vi "Configure Library Classes in Memory for Build.vi"(5 "custom class options":T1[](array[typedef]), 7 "target name (My Computer)":string="My Computer", 9 "enable debug? (F)":bool, 10 "save VIs? (T)":bool=TRUE, 11 "library name":string="DSF Core.lvlib") -> (0 "error out":errorcluster)   [LabVIEW 2017, in "Build Automation.lvlib"]
uses:
  Build Automation.lvlib
  Class VI Options.ctl
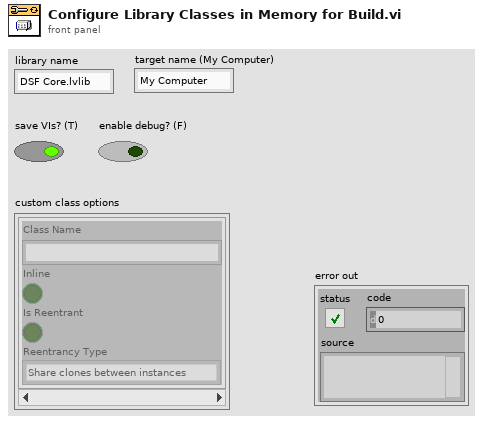
[diagram p1: front panel]
types:
  T1 = typedef "Build Automation.lvlib/Class VI Options.ctl" = cluster{"Class Name":string, "Inline":bool, "Is Reentrant":bool, "Reentrancy Type":enum16{"Share clones between instances", "Preallocate clone for each instance"}}
  T2 = cluster{"Status Message":refnum<data-value>, "Progress":refnum<data-value>, "Stop":refnum<data-value>}
  T3 = enum16{"Share clones between instances", "Preallocate clone for each instance"}
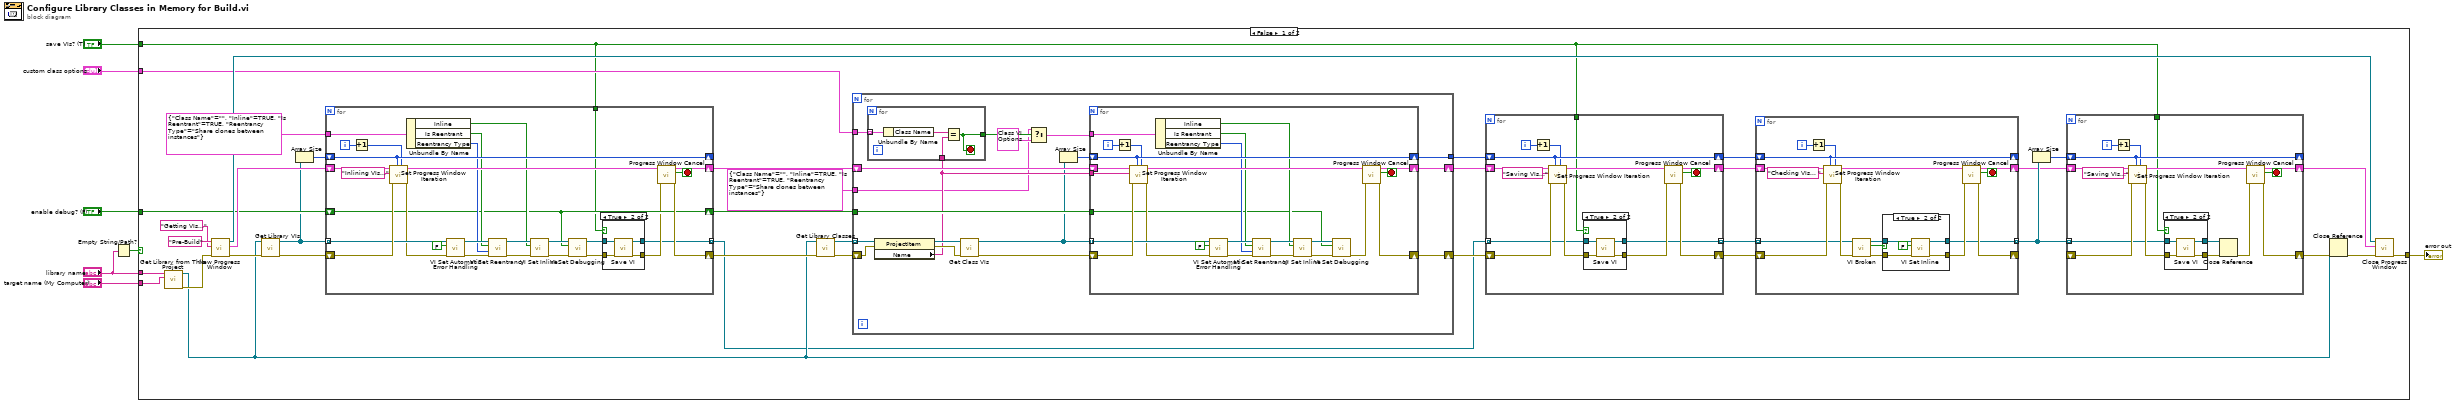
[diagram p0: block diagram]
diagram:
  n1 = Empty String/Path?(string/path="library name") -> (empty?=w6:bool)
  n2 = case shown="False" w6 {
    tunnel: [w43 _] -> w4
    tunnel: "enable debug? (F)" -> [w25 _]
    tunnel: "library name" -> [w38 _]
    tunnel: "save VIs? (T)" -> [w8 _]
    tunnel: "target name (My Computer)" -> [w36 _]
    tunnel: "custom class options" -> [w23 _]
    frame False {
      n3 = call "Get Library from This Project.vi"("Target Name (My Computer)"=w36, "Library Name"=w38) -> ("error out"=w37:errorcluster, "Library Refnum"=w27:refnum<vi>)  [unwired: 8 in]
      n4 = call "New Progress Window.vi"("error in (no error)"=w37, "Initial Message"="Getting VIs...", "Window Title"="Pre-Build" ("WindowTitle")) -> ("error out"=w28:errorcluster, "DVRs"=w29:T2, "VI refnum"=w44:refnum<vi>)  [unwired: 6 in]
      n5 = call "Get Library VIs.vi"("error in (no error)"=w28, "library ref"=w27) -> ("error out"=w26:errorcluster, "vi refs"=w21:refnum<vi>[])  [unwired: 8 in]
      n6 = Array Size(array=w21) -> (size(s)=w22:i32)
      n7 = for {
        tunnel: w21 -> [w64] mode=indexing
        shift-right: [w71] -> w31
        shift-left: w29 -> [w68]
        shift-right: [w65] -> w30
        shift-left: w26 -> [w66]
        tunnel: [w45] -> w11 mode=indexing
        shift-right: [w63] -> _
        shift-left: w22 -> [w63]
        tunnel: T1 {"Class Name"="", "Inline"=TRUE, "Is Reentrant"=TRUE, "Reentrancy Type"=enum."Share clones between instances"} ("f") -> [w56]
        shift-right: [w51] -> w24
        shift-left: w25 -> [w51]
        tunnel: w8 -> [w46]
        i -> [w73]
        stop <- w72 stop-if-true
        n8 = Increment(x=w73) -> (x+1=w62:i32)
        n9 = call "Set Progress Window Iteration.vi"("current iteration"=w62, "total iterations"=w63, "error in (no error)"=w66, "Status Message"="Inlining VIs...", "DVRs in"=w68) -> ("error out"=w53:errorcluster, "DVRs out"=w67:T2)  [unwired: 5 in]
        n10 = Unbundle By Name(w56) -> ("Inline"=w55:bool, "Is Reentrant"=w54:bool, "Reentrancy Type"=w52:T3)
        n11 = call "VI Set Automatic Error Handling.vi"("error in (no error)"=w53, "Automatic Error Handling"=FALSE, "vi ref in"=w64) -> ("error out"=w57:errorcluster, "vi ref out"=w69:refnum<vi>)  [unwired: 7 in]
        n12 = call "VI Set Reentrancy.vi"("error in (no error)"=w57, "Reentrancy Type (shared clone)"=w52, "Is Reentrant"=w54, "vi ref in"=w69) -> ("error out"=w60:errorcluster, "vi ref out"=w61:refnum<vi>)  [unwired: 6 in]
        n13 = call "VI Set Inline.vi"("error in (no error)"=w60, "Inline VI"=w55, "vi ref in"=w61) -> ("error out"=w58:errorcluster, "vi ref out"=w59:refnum<vi>)  [unwired: 7 in]
        n14 = call "VI Set Debugging.vi"("error in (no error)"=w58, "Allow Debugging"=w51, "vi ref in"=w59) -> ("error out"=w48:errorcluster, "vi ref out"=w49:refnum<vi>)  [unwired: 7 in]
        n15 = case shown="True" w46 {
          tunnel: w48 -> [w74 w79]
          tunnel: [w75 w78] -> w45
          tunnel: [w74 w77] -> w47
          tunnel: w49 -> [w75 w76]
          frame False {
          }
          frame True {
            n16 = call "Save VI.vi"("error in (no error)"=w79, "vi ref in"=w76) -> ("error out"=w77:errorcluster, "vi ref out"=w78:refnum<vi>)  [unwired: 8 in]
          }
        }
        n17 = call "Progress Window Cancel.vi"("error in (no error)"=w47, "DVRs in"=w67) -> ("error out"=w65:errorcluster, "cancelled"=w72:bool, "DVRs out"=w71:T2)  [unwired: 7 in]
      }
      n18 = call "Get Library Classes.vi"("error in (no error)"=w30, "library ref"=w27) -> ("error out"=w34:errorcluster, "class refs"=w33:refnum<vi>[])  [unwired: 8 in]
      n19 = for {
        tunnel: w24 -> [w96]
        tunnel: [w94] -> w15
        tunnel: w33 -> [w90] mode=indexing
        shift-right: [w92] -> w17
        shift-left: w34 -> [w88]
        shift-right: [w93] -> w16
        shift-left: w31 -> [w97]
        tunnel: w23 -> [w81]
        tunnel: T1 {"Class Name"="", "Inline"=TRUE, "Is Reentrant"=TRUE, "Reentrancy Type"=enum."Share clones between instances"} ("f") -> [w80]
        n20 = property class="ProjectItem"(reference=w90, error in=w88) -> (reference out=w89:refnum<vi>, error out=w87:errorcluster, "Name"=w86:string)
        n21 = for {
          tunnel: w86 -> [w101]
          tunnel: [w100] -> w85
          tunnel: w81 -> [w99] mode=indexing
          stop <- w100 stop-if-true
          n22 = Unbundle By Name(w99) -> ("Class Name"=w98:string)
          n23 = Equal?(x=w98, y=w101) -> (x = y?=w100:bool)
        }
        n24 = call "Get Class VIs.vi"("error in (no error)"=w87, "class ref"=w89) -> ("error out"=w91:errorcluster, "vi refs"=w82:refnum<vi>[])  [unwired: 8 in]
        n25 = Select(t=w80, s=w85, f=T1 {"Class Name"="", "Inline"=FALSE, "Is Reentrant"=FALSE, "Reentrancy Type"=enum."Share clones between instances"}) -> (s? t:f=w83:T1)
        n26 = Array Size(array=w82) -> (size(s)=w95:i32)
        n27 = for {
          tunnel: w82 -> [w117] mode=indexing
          shift-right: [w124] -> w93
          shift-left: w97 -> [w121]
          shift-right: [w118] -> w92
          shift-left: w91 -> [w119]
          tunnel: w96 -> [w102]
          shift-right: [w116] -> w94
          shift-left: w95 -> [w116]
          tunnel: w86 -> [w108]
          tunnel: w83 -> [w107]
          i -> [w126]
          stop <- w125 stop-if-true
          n28 = Increment(x=w126) -> (x+1=w115:i32)
          n29 = call "Set Progress Window Iteration.vi"("current iteration"=w115, "total iterations"=w116, "error in (no error)"=w119, "Status Message"=w108, "DVRs in"=w121) -> ("error out"=w104:errorcluster, "DVRs out"=w120:T2)  [unwired: 5 in]
          n30 = Unbundle By Name(w107) -> ("Inline"=w106:bool, "Is Reentrant"=w105:bool, "Reentrancy Type"=w103:T3)
          n31 = call "VI Set Automatic Error Handling.vi"("error in (no error)"=w104, "Automatic Error Handling"=FALSE, "vi ref in"=w117) -> ("error out"=w109:errorcluster, "vi ref out"=w122:refnum<vi>)  [unwired: 7 in]
          n32 = call "VI Set Reentrancy.vi"("error in (no error)"=w109, "Reentrancy Type (shared clone)"=w103, "Is Reentrant"=w105, "vi ref in"=w122) -> ("error out"=w113:errorcluster, "vi ref out"=w114:refnum<vi>)  [unwired: 6 in]
          n33 = call "VI Set Inline.vi"("error in (no error)"=w113, "Inline VI"=w106, "vi ref in"=w114) -> ("error out"=w111:errorcluster, "vi ref out"=w112:refnum<vi>)  [unwired: 7 in]
          n34 = call "VI Set Debugging.vi"("error in (no error)"=w111, "Allow Debugging"=w102, "vi ref in"=w112) -> ("error out"=w110:errorcluster)  [unwired: 7 in, 1 out]
          n35 = call "Progress Window Cancel.vi"("error in (no error)"=w110, "DVRs in"=w120) -> ("error out"=w118:errorcluster, "cancelled"=w125:bool, "DVRs out"=w124:T2)  [unwired: 7 in]
        }
      }
      n36 = for {
        tunnel: w11 -> [w129] mode=indexing
        shift-right: [w139] -> w13
        shift-left: w16 -> [w138]
        shift-right: [w135] -> w12
        shift-left: w17 -> [w136]
        shift-right: [w134] -> w14
        shift-left: w15 -> [w134]
        tunnel: w8 -> [w128]
        tunnel: [w127] -> w10 mode=indexing
        i -> [w141]
        stop <- w140 stop-if-true
        n37 = Increment(x=w141) -> (x+1=w133:i32)
        n38 = call "Set Progress Window Iteration.vi"("current iteration"=w133, "total iterations"=w134, "error in (no error)"=w136, "Status Message"="Saving VIs...", "DVRs in"=w138) -> ("error out"=w131:errorcluster, "DVRs out"=w137:T2)  [unwired: 5 in]
        n39 = case shown="True" w128 {
          tunnel: w131 -> [w142 w147]
          tunnel: [w143 w146] -> w127
          tunnel: [w142 w145] -> w130
          tunnel: w129 -> [w143 w144]
          frame False {
          }
          frame True {
            n40 = call "Save VI.vi"("error in (no error)"=w147, "vi ref in"=w144) -> ("error out"=w145:errorcluster, "vi ref out"=w146:refnum<vi>)  [unwired: 8 in]
          }
        }
        n41 = call "Progress Window Cancel.vi"("error in (no error)"=w130, "DVRs in"=w137) -> ("error out"=w135:errorcluster, "cancelled"=w140:bool, "DVRs out"=w139:T2)  [unwired: 7 in]
      }
      n42 = for {
        tunnel: w10 -> [w153] mode=indexing
        shift-right: [w162] -> w9
        shift-left: w13 -> [w161]
        shift-right: [w158] -> _
        shift-left: w12 -> [w159]
        shift-right: [w157] -> _
        shift-left: w14 -> [w157]
        tunnel: [w148] -> w18 mode=indexing
        i -> [w164]
        stop <- w163 stop-if-true
        n43 = Increment(x=w164) -> (x+1=w156:i32)
        n44 = call "Set Progress Window Iteration.vi"("current iteration"=w156, "total iterations"=w157, "error in (no error)"=w159, "Status Message"="Checking VIs... ", "DVRs in"=w161) -> ("error out"=w154:errorcluster, "DVRs out"=w160:T2)  [unwired: 5 in]
        n45 = call "VI Broken.vi"("error in (no error)"=w154, "vi ref in"=w153) -> ("error out"=w151:errorcluster, "broken?"=w150:bool, "vi ref out"=w152:refnum<vi>)  [unwired: 7 in]
        n46 = case shown="True" w150 {
          tunnel: [w166 w171] -> w148
          tunnel: [w165 w170] -> w149
          tunnel: w151 -> [w165 w169]
          tunnel: w152 -> [w166 w167]
          frame False {
          }
          frame True {
            n47 = call "VI Set Inline.vi"("error in (no error)"=w169, "Inline VI"=FALSE, "vi ref in"=w167) -> ("error out"=w170:errorcluster, "vi ref out"=w171:refnum<vi>)  [unwired: 7 in]
          }
        }
        n48 = call "Progress Window Cancel.vi"("error in (no error)"=w149, "DVRs in"=w160) -> ("error out"=w158:errorcluster, "cancelled"=w163:bool, "DVRs out"=w162:T2)  [unwired: 7 in]
      }
      n49 = Array Size(array=w18) -> (size(s)=w32:i32)
      n50 = for {
        tunnel: w18 -> [w173] mode=indexing
        shift-right: [w185] -> w42
        shift-left: w9 -> [w184]
        shift-right: [w181] -> w40
        shift-left: _ -> [w182]
        shift-right: [w180] -> _
        shift-left: w32 -> [w180]
        tunnel: w8 -> [w172]
        i -> [w187]
        stop <- w186 stop-if-true
        n51 = Increment(x=w187) -> (x+1=w179:i32)
        n52 = call "Set Progress Window Iteration.vi"("current iteration"=w179, "total iterations"=w180, "error in (no error)"=w182, "Status Message"="Saving VIs...", "DVRs in"=w184) -> ("error out"=w177:errorcluster, "DVRs out"=w183:T2)  [unwired: 5 in]
        n53 = case shown="True" w172 {
          tunnel: w177 -> [w188 w193]
          tunnel: [w189 w192] -> w176
          tunnel: [w188 w191] -> w175
          tunnel: w173 -> [w189 w190]
          frame False {
          }
          frame True {
            n54 = call "Save VI.vi"("error in (no error)"=w193, "vi ref in"=w190) -> ("error out"=w191:errorcluster, "vi ref out"=w192:refnum<vi>)  [unwired: 8 in]
          }
        }
        n55 = Close Reference(reference=w176, error in (no error)=w175) -> (error out=w174:errorcluster)
        n56 = call "Progress Window Cancel.vi"("error in (no error)"=w174, "DVRs in"=w183) -> ("error out"=w181:errorcluster, "cancelled"=w186:bool, "DVRs out"=w185:T2)  [unwired: 7 in]
      }
      n57 = Close Reference(reference=w27, error in (no error)=w40) -> (error out=w39:errorcluster)
      n58 = call "Close Progress Window.vi"("error in (no error)"=w39, "DVRs in"=w42, "VI refnum"=w44) -> ("error out"=w43:errorcluster)  [unwired: 8 in]
    }
    frame True {
    }
  }
  "error out" <- w4
